vi "crashdetect_overview.vi"   [LabVIEW 2015]
doc: "Update global variable indicating whether the aircraft has crashed.\nThe aircraft is determined to have crashed if it exceed 5g gravity at any time."
uses:
  global.vi
types:
  T1 = cluster{"Airspeed":dbl, "Altitude":dbl, "Vertical Speed":dbl, "Pitch":dbl, "Roll":dbl, "Heading":dbl, "Turn Indicator":dbl, "Latitude":dbl, "Longitude":dbl, "pilot g":dbl, "view number":i16, "fov":dbl, "view heading":dbl, "view pitch":dbl, "game width":i16, "game height":i16}
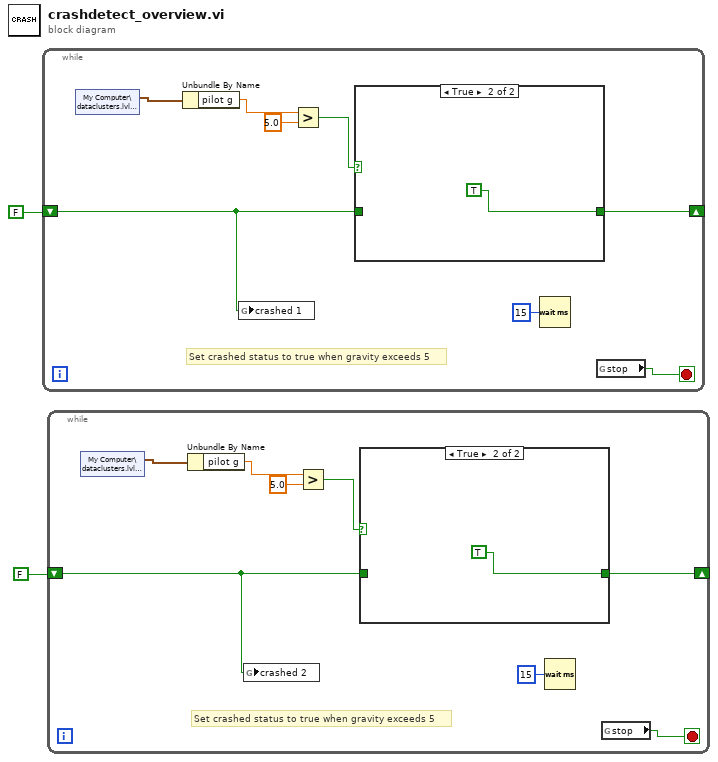
[diagram p0: block diagram]
diagram:
  n1 = while {
    shift-right: [w7] -> _
    shift-left: FALSE -> [w6]
    stop <- w5 stop-if-true
    # "Set crashed status to true when gravity exceeds 5"
    n2 = shared-variable "My Computer\\dataclusters.lvlib\\pc1"() -> (w4:T1)  [unwired: 1 in, 1 out]
    n3 = Unbundle By Name(w4) -> ("pilot g"=w10:dbl)
    n4 = global write "global.vi" "crashed 1"(w6) -> ()
    n5 = Greater?(x=w10, y=5.0) -> (0:w8:bool)
    n6 = case shown="True" w8 {
      tunnel: w6 -> [w11 _]
      tunnel: [w11 TRUE] -> w7
      frame False {
      }
      frame True {
      }
    }
    n7 = Wait (ms)(milliseconds to wait=u32 15) -> ()  [unwired: 1 out]
    n8 = global read "global.vi" "stop"() -> (w5:bool)
  }
  n9 = while {
    shift-right: [w17] -> _
    shift-left: FALSE -> [w16]
    stop <- w15 stop-if-true
    # "Set crashed status to true when gravity exceeds 5"
    n10 = shared-variable "My Computer\\dataclusters.lvlib\\pc2"() -> (w14:T1)  [unwired: 1 in, 1 out]
    n11 = Unbundle By Name(w14) -> ("pilot g"=w20:dbl)
    n12 = global write "global.vi" "crashed 2"(w16) -> ()
    n13 = Greater?(x=w20, y=5.0) -> (0:w18:bool)
    n14 = case shown="True" w18 {
      tunnel: w16 -> [w21 _]
      tunnel: [w21 TRUE] -> w17
      frame False {
      }
      frame True {
      }
    }
    n15 = Wait (ms)(milliseconds to wait=u32 15) -> ()  [unwired: 1 out]
    n16 = global read "global.vi" "stop"() -> (w15:bool)
  }
